vi "Manipulate Auto Velocities.vi"(8 "Zero Translational V":bool, 9 "Zero V":bool, 10 "Position":cluster{"x":dbl, "y":dbl, "th":dbl}, 11 "Robot Velocities":T2) -> (1 "Done?":bool, 2 "Drive Conditions":T1, 3 "Robot Velocities Out":T2)   [LabVIEW 2025]
uses:
  swerve-template/Type Definitions/Data/Robot Velocities.ctl
  Framework/Drive Conditions.ctl
  Framework/Robot Global Data.vi
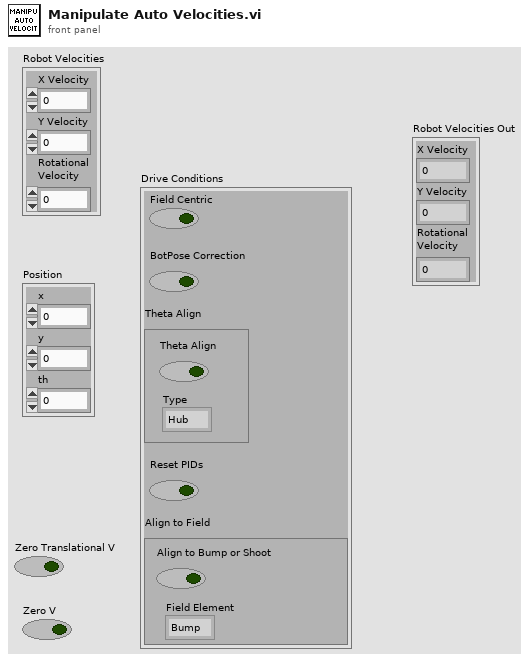
[diagram p1: front panel]
types:
  T1 = typedef "Drive Conditions.ctl" = cluster{"Field Centric":bool, "BotPose Correction":bool, "Theta Align":cluster{"Theta Align":bool, "Type":enum16{"Hub", "Corner of Field"}}, "Reset PIDs":bool, "Align to Field":cluster{"Align to Bump or Shoot":bool, "Field Element":enum16{"Bump", "Shooter Shot", "Trench"}}}
  T2 = typedef "Robot Velocities.ctl" = cluster{"X Velocity":dbl, "Y Velocity":dbl, "Rotational \nVelocity":dbl}
  T3 = cluster{"Theta Align":bool, "Type":enum16{"Hub", "Corner of Field"}}
  T4 = cluster{"Align to Bump or Shoot":bool, "Field Element":enum16{"Bump", "Shooter Shot", "Trench"}}
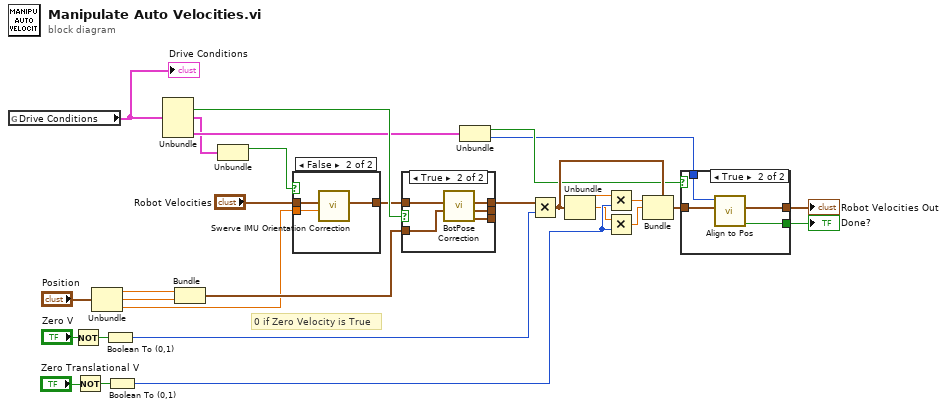
[diagram p0: block diagram]
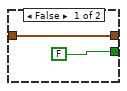
[diagram p4: hidden frame]
diagram:
  # "0 if Zero Velocity is True"
  n1 = global read "Robot Global Data.vi" "Drive Conditions"() -> (w24:T1)
  "Drive Conditions" <- w24
  n2 = Not(x="Zero V") -> (.not. x?=w16:bool)
  n3 = Not(x="Zero Translational V") -> (.not. x?=w14:bool)
  n4 = Unbundle("Position") -> ("x"=w21:dbl, "y"=w22:dbl, "th"=w19:dbl)
  n5 = Boolean To (0,1)(Boolean=w16) -> (0, 1=w17:i16)
  n6 = Boolean To (0,1)(Boolean=w14) -> (0, 1=w12:i16)
  n7 = Unbundle(w24) -> ("BotPose Correction"=w25:bool, "Theta Align"=w2:T3, "Align to Field"=w5:T4)  [unwired: 2 out]
  n8 = Bundle("x"=w21, "y"=w22) -> (w23:cluster{"x":dbl, "y":dbl})  [unwired: 1 in]
  n9 = Unbundle(w2) -> ("Theta Align"=w1:bool)  [unwired: 1 out]
  n10 = case shown="False" w1 {
    tunnel: w19 -> [_ w33]
    tunnel: [w30 w32] -> w20
    tunnel: "Robot Velocities" -> [w30 w31]
    frame True {
    }
    frame False {
      n11 = call "Swerve IMU Orientation Correction.vi"("Setpoint"=w33, "Robot Velocities In"=w31) -> ("Robot Velocities Out"=w32:T2)  [unwired: 9 in]
    }
  }
  n12 = case shown="True" w25 {
    tunnel: w20 -> [w34 w39]
    tunnel: [w34 w38] -> w28
    tunnel: w23 -> [_ w37]
    tunnel: [_ w36] -> _
    tunnel: [_ w35] -> _
    frame False {
    }
    frame True {
      n13 = call "BotPose Correction.vi"("Pos In"=w37, "Robot Velocities In"=w39) -> ("BotPose"=w35:cluster{"Numeric":dbl, "Numeric":dbl}, "Bordeaux Pos"=w36:cluster{dbl, dbl}, "Robot Velocities Out"=w38:T2)  [unwired: 7 in]
    }
  }
  n14 = Unbundle(w5) -> ("Align to Bump or Shoot"=w4:bool, "Field Element"=w3:enum16{"Bump", "Shooter Shot", "Trench"})
  n15 = Multiply(x=w28, y=w17) -> (x*y=w6:T2)
  n16 = Unbundle(w6) -> ("X Velocity"=w10:dbl, "Y Velocity"=w11:dbl)  [unwired: 1 out]
  n17 = Multiply(x=w10, y=w12) -> (x*y=w9:dbl)
  n18 = Multiply(x=w11, y=w12) -> (x*y=w8:dbl)
  n19 = Bundle(cluster=w6, "X Velocity"=w9, "Y Velocity"=w8) -> (w7:T2)  [unwired: 1 in]
  n20 = case shown="True" w4 {
    tunnel: [w41 w45] -> w27
    tunnel: w7 -> [w41 w44]
    tunnel: [FALSE ("Done?") w43] -> w29
    tunnel: w3 -> [_ w42]
    frame False {
    }
    frame True {
      n21 = call "Align to Pos.vi"("Robot Velocities In"=w44, "Field Element"=w42) -> ("Done?"=w43:bool, "Robot Velocities Out"=w45:T2)  [unwired: 8 in]
    }
  }
  "Done?" <- w29
  "Robot Velocities Out" <- w27
